vi "add or sub waveforms.vi"(7 "operation":bool, 8 "inf":dbl=-10.0 format="%#_13g", 9 "Waveform 2":waveform(dbl), 10 "Waveform 1":waveform(dbl), 11 "sup":dbl=10.0 format="%#_13g") -> (2 "New Waveform":waveform(dbl))   [LabVIEW 2019]
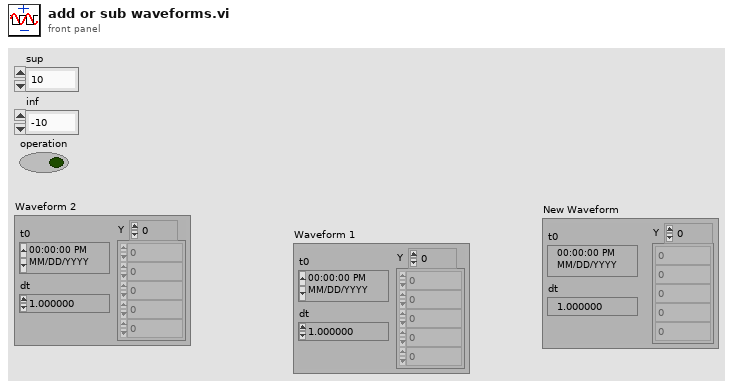
[diagram p1: front panel]
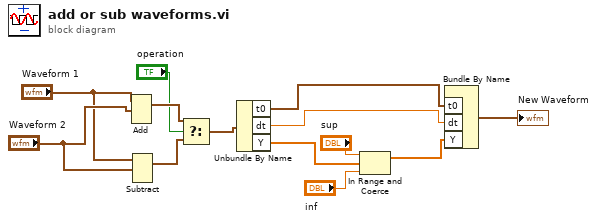
[diagram p0: block diagram]
diagram:
  n1 = Add(1:"Waveform 2", 2:"Waveform 1") -> (0:w6:waveform(dbl))  [unwired: 1 in, 1 out]
  n2 = Subtract(1:"Waveform 2", 2:"Waveform 1") -> (0:w5:waveform(dbl))  [unwired: 1 in, 1 out]
  n3 = Select(t=w6, s="operation", f=w5) -> (s? t:f=w7:waveform(dbl))
  n4 = Unbundle By Name(w7) -> ("t0"=w8:timestamp, "dt"=w11:dbl, "Y"=w13:dbl[])
  n5 = In Range and Coerce(upper limit="sup", x=w13, lower limit="inf") -> (coerced(x)=w12:dbl[])  [unwired: 1 out]
  n6 = Bundle By Name("t0"=w8, "dt"=w11, "Y"=w12) -> (→"New Waveform":waveform(dbl))  [unwired: 1 in]
